vi "ifr2025 Sinad.vi"(5 "Delta Level Step (1.0)":dbl=1.0, 6 "Auto Target (12.0)":dbl=12.0, 7 "Mode (Disable)":i16(ring) items=["Disable", "Enable", "Auto"], 8 "error in (no error)":errorcluster {"code" format="%.0x"}, 9 "Filter Weighting (C-MESS)":i16(ring)=2 items=["None", "CCITT", "C-MESS"], 10 "Averages (0)":i32 min=1 max=127 step=1 format="%.0g", 11 "instrument handle":refnum<visa-resource-name>) -> (0 "error out":errorcluster {"code" format="%.0x"}, 3 "instrument handle out":refnum<visa-resource-name>)   [LabVIEW 2009]
doc: "This function allows the parameters relating to Sinad measurement to be specified.\nIf Mode AUTO is selected then an 'Auto Target' value should be specified."
uses:
  Ifr2025_32.dll
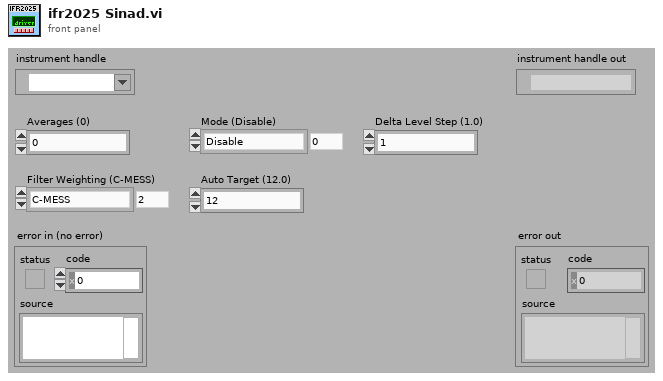
[diagram p1: front panel]
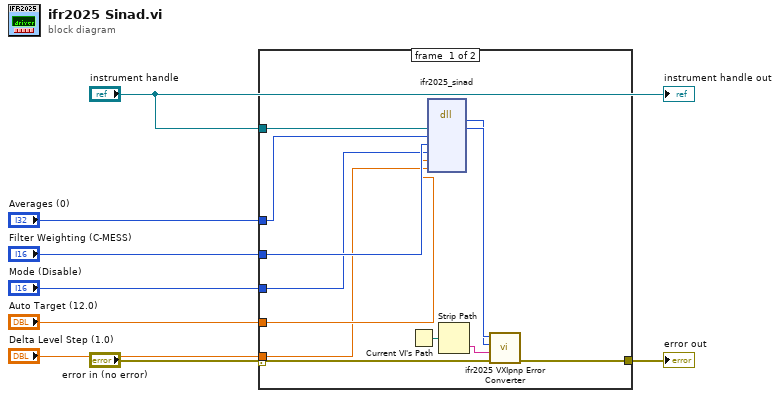
[diagram p0: block diagram]
diagram:
  n1 = case shown="No Error" "error in (no error)" {
    selector: "error in (no error)" -> [w15 w21]
    tunnel: [w14 w21] -> w8
    tunnel: "instrument handle" -> [w19 _]
    tunnel: "Averages (0)" -> [w13 _]
    tunnel: "Filter Weighting (C-MESS)" -> [w12 _]
    tunnel: "Mode (Disable)" -> [w11 _]
    tunnel: "Auto Target (12.0)" -> [w10 _]
    tunnel: "Delta Level Step (1.0)" -> [w9 _]
    frame #0 {
      n2 = Current VI's Path() -> (path=w20:path)
      n3 = dll-call lib="P:/inst/Marconi 2024 Signal Generator/source/labview/ifr2025/ifr2025/ifr2025_*.*" fn="ifr2025_sinad"("vi"=w19, "Averages"=w13, "Filter Weighting"=w12, "Mode"=w11, "Auto Target"=w10, "Delta Level Step"=w9) -> (w17:i32, "vi"=w18:u32)  [unwired: 8 in, 2 out]
      n4 = Strip Path(path=w20) -> (name=w16:string)  [unwired: 1 out]
      n5 = call "ifr2025 VXIpnp Error Converter.vi"("error in (no error)"=w15, "name of VI (\"\")"=w16, "CVI error code (0)"=w17, "instrument handle"=w18) -> ("error out"=w14:errorcluster)  [unwired: 7 out]
    }
    frame #1 {
    }
  }
  "error out" <- w8
  "instrument handle out" <- "instrument handle"
